vi "Open.vi"(8 "error in (no error)":errorcluster, 11 "subprocess in":refnum<class "Buffered Subprocess.lvclass">) -> (0 "error out":errorcluster, 3 "subprocess out":refnum<class "Buffered Subprocess.lvclass">)   [LabVIEW 2020, in "NI_Subprocess.lvlib" / "Buffered Subprocess.lvclass"]
uses:
  <vilib>/Subprocess/Buffered Subprocess/Buffered Subprocess.lvclass
  <vilib>/Subprocess/Buffered Subprocess/Buffered Subprocess.lvclass/Buffered Subprocess.ctl
  <vilib>/Subprocess/Subprocess/Subprocess.lvclass
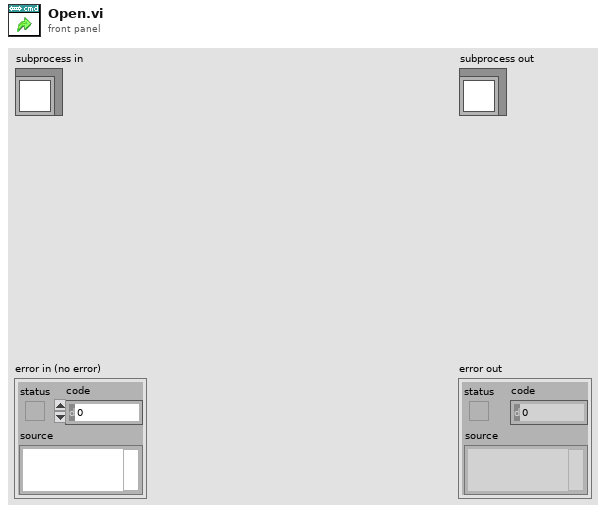
[diagram p1: front panel]
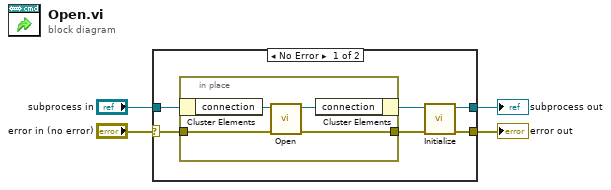
[diagram p0: block diagram]
diagram:
  n1 = case shown="No Error" "error in (no error)" {
    selector: "error in (no error)" -> [w9 w16]
    tunnel: [w5 w16] -> w3
    tunnel: [w6 w15] -> w1
    tunnel: "subprocess in" -> [w10 w15]
    frame No Error {
      n2 = in-place {
        in-place-border: w9 -> [w12]
        in-place-border: [w11] -> w7
        n3 = in-place-cluster #1(w10) -> ("connection"=w14:refnum<class "Subprocess.lvclass">)
        n4 = call <vilib>:"Open.vi"("error in (no error)"=w12, "subprocess in"=w14) -> ("error out"=w11:errorcluster, "subprocess out"=w13:refnum<class "Subprocess.lvclass">)  [unwired: 8 in]
        n5 = in-place-cluster #1("connection"=w13) -> (w8:refnum<class "Buffered Subprocess.lvclass">)
      }
      n6 = call-dynamic "Initialize.vi"("error in (no error)"=w7, "subprocess in"=w8) -> ("error out"=w5:errorcluster, "subprocess out"=w6:refnum<class "Buffered Subprocess.lvclass">)  [unwired: 8 in]
    }
    frame Error {
    }
  }
  "error out" <- w3
  "subprocess out" <- w1
